vi "Load-sequences-from-file.vi"(8 "error in (no error)":errorcluster, 10 "Path":path, 11 "Available motors in":refnum<class "Motor-assembly.lvclass">) -> (0 "error out":errorcluster, 3 "Available motors out":refnum<class "Motor-assembly.lvclass">)   [LabVIEW 2013, in "PowderDeposition.lvlib" / "Motor-assembly.lvclass"]
uses:
  Motor-assembly.lvclass
  Motor-assembly.lvclass/Motor-assembly.ctl
  Motor/Motor.lvclass
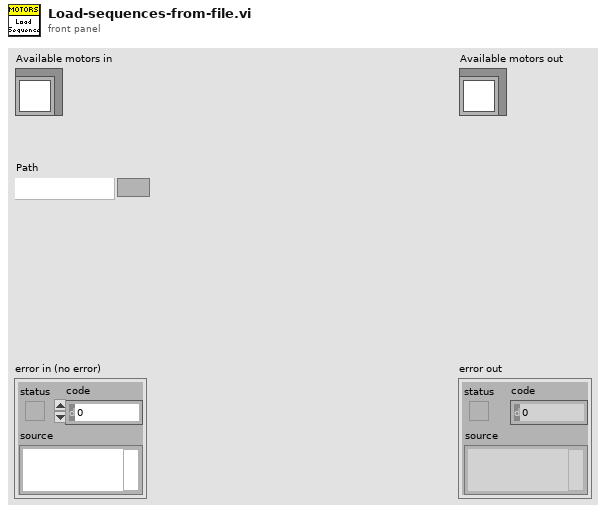
[diagram p1: front panel]
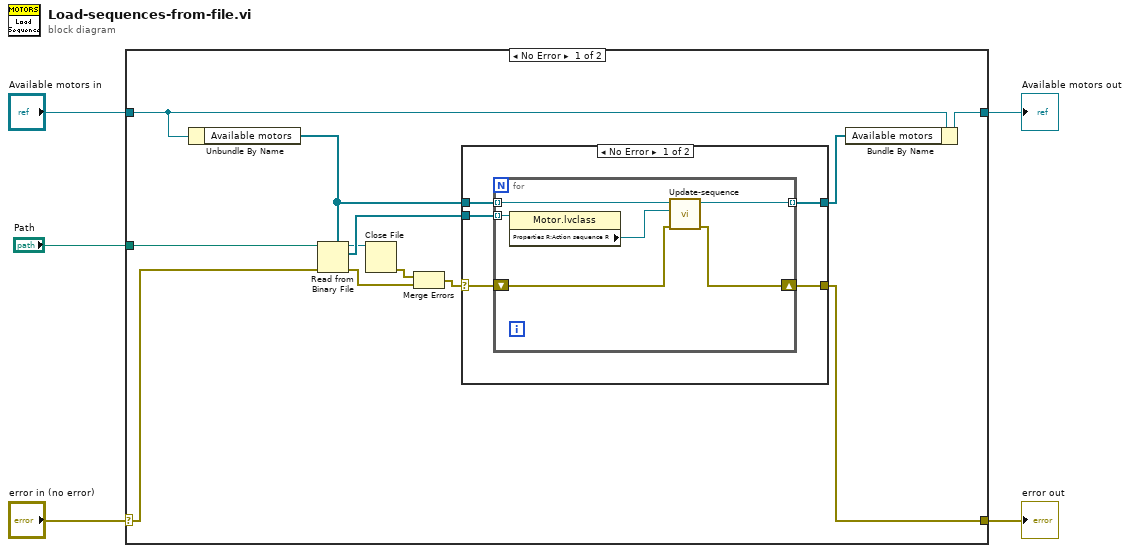
[diagram p0: block diagram]
diagram:
  n1 = case shown="No Error" "error in (no error)" {
    selector: "error in (no error)" -> [w15 w32]
    tunnel: [w7 w32] -> w4
    tunnel: [w16 w31] -> w2
    tunnel: "Available motors in" -> [w17 w31]
    tunnel: "Path" -> [w14 _]
    frame No Error {
      n2 = Unbundle By Name(w17) -> ("Available motors"=w9:refnum<class "Motor.lvclass">[])
      n3 = Read from Binary File(5:w9, 8:w15, 11:w14) -> (0:w11:errorcluster, 2:w10:refnum<class "Motor.lvclass">[], 3:w6:refnum<file>)  [unwired: 3 in, 1 out]
      n4 = Close File(refnum=w6) -> (error out=w12:errorcluster)  [unwired: 1 in, 1 out]
      n5 = Merge Errors(w12, w11) -> (w8:errorcluster)
      n6 = case shown="No Error" w8 {
        selector: w8 -> [w18 w29]
        tunnel: w9 -> [w22 w30]
        tunnel: w10 -> [w21 _]
        tunnel: [w20 w30] -> w13
        tunnel: [w19 w29] -> w7
        frame No Error {
          n7 = for {
            tunnel: w21 -> [w28] mode=indexing
            tunnel: w22 -> [w27] mode=indexing
            tunnel: [w25] -> w20 mode=indexing
            shift-right: [w23] -> w19
            shift-left: w18 -> [w24]
            n8 = property class="Motor.lvclass"(reference=w28) -> ("Properties R:Action sequence R"=w26:refnum<class "Action-sequence.lvclass">)  [unwired: 1 in, 2 out]
            n9 = call-dynamic "Update-sequence.vi"("error in (no error)"=w24, "Sequence"=w26, "Motor in"=w27) -> ("error out"=w23:errorcluster, "Motor out"=w25:refnum<class "Motor.lvclass">)  [unwired: 7 in]
          }
        }
        frame Error {
        }
      }
      n10 = Bundle By Name(cluster=w17, "Available motors"=w13) -> (w16:refnum<class "Motor-assembly.lvclass">)
    }
    frame Error {
    }
  }
  "error out" <- w4
  "Available motors out" <- w2
